vi "is-1.vi"(4 "Value":i32) -> (1 "is -1?":bool)   [LabVIEW 2017]
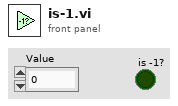
[diagram p1: front panel]
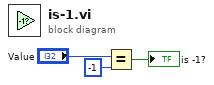
[diagram p0: block diagram]
diagram:
  n1 = Equal?(x="Value", y=-1) -> (x = y?=→"is -1?":bool)
